vi "DAC_current_values.vi"(1 "FPGA Ref":T1) -> (0 "DAC values":sgl[][](array[numeric]))   [LabVIEW 2013]
uses:
  fpga-bitfile-ref.ctl
  <vilib>/Utility/error.llb/Error Cluster From Error Code.vi
  <vilib>/rvi/errors/niLvFpgaAdjustHostInterfaceError.vi
  <vilib>/rvi/interface/nirviReadWriteControl/nirviReadWriteControl.xnode
  FPGA Bitfiles/fpga-clean1_FPGATarget_FPGAMAINlock-in_FC21E42C.lvbitx
  NiFpgaLv.dll
panel:
  in  "exit":bool
  out "FPGA VI Reference":T1
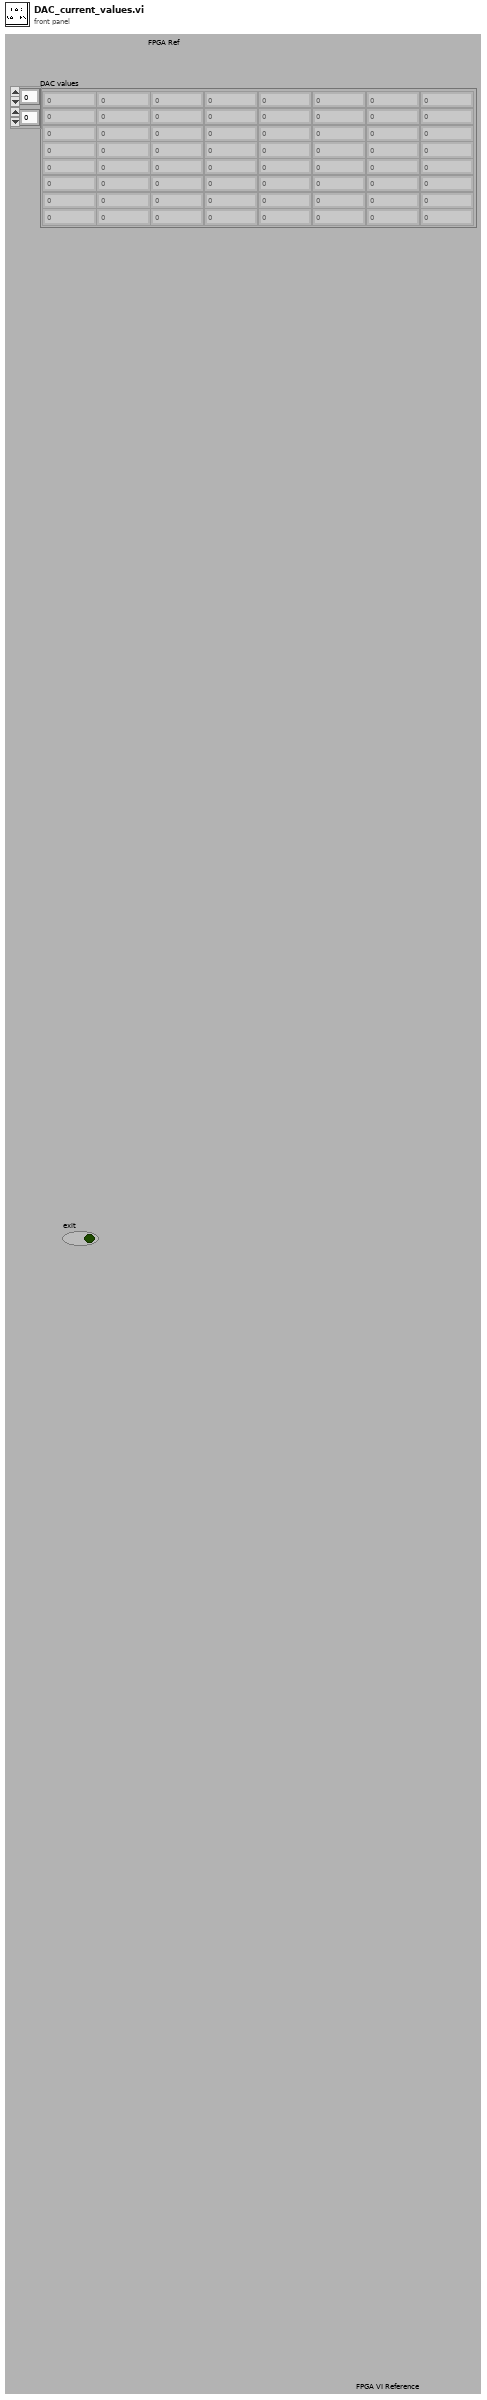
[diagram p1: front panel]
types:
  T1 = typedef "fpga-bitfile-ref.ctl" = refnum<k20>
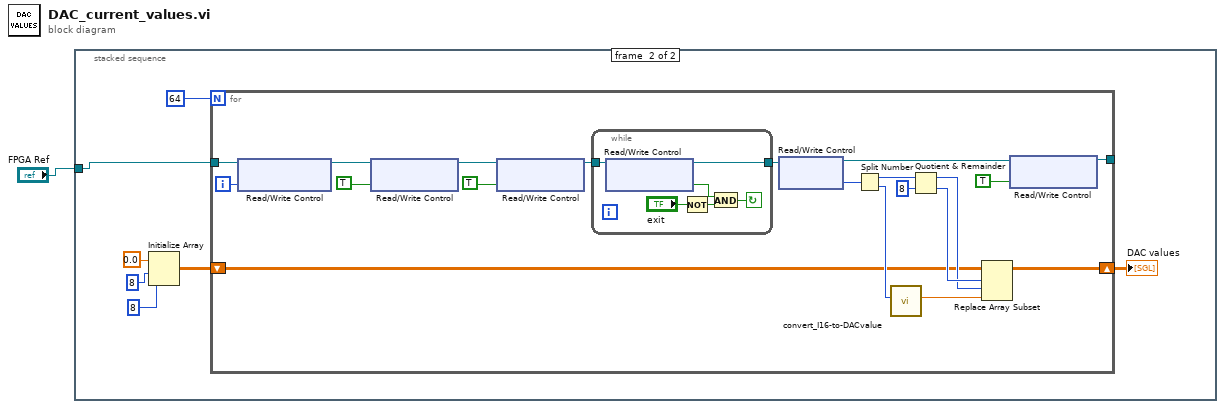
[diagram p0: block diagram]
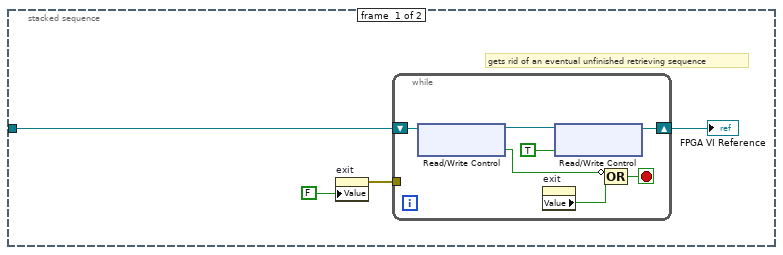
[diagram p2: hidden frame]
diagram:
  n1 = stacked-sequence {
    tunnel: "FPGA Ref" -> [w2 w18]
    frame #0 {
      # "gets rid of an eventual unfinished retrieving sequence"
      n2 = property on="exit" class="Bool (strict)"("Value"=FALSE ("exit")) -> (error out=w4:errorcluster)  [unwired: 2 in, 1 out]
      n3 = while {
        shift-right: [w10] -> w3
        shift-left: w2 -> [w12]
        tunnel: w4 -> [_]
        stop <- w8 stop-if-true
        n4 = xnode "Read/Write Control"("FPGA VI Reference In"=w12) -> ("FPGA VI Reference Out"=w11:T1, "get DAC value"=w7:bool)  [unwired: 1 in, 1 out]
        n5 = property on="exit" class="Bool (strict)"() -> ("Value"=w9:bool)  [unwired: 2 in, 2 out]
        n6 = xnode "Read/Write Control"("FPGA VI Reference In"=w11, "got DAC value"=TRUE) -> ("FPGA VI Reference Out"=w10:T1)  [unwired: 1 in, 1 out]
        n7 = Compound Arithmetic op=OR(invert w7, w9) -> (w8:bool)
      }
      "FPGA VI Reference" <- w3
    }
    frame #1 {
      n8 = Initialize Array(0.0, 8, 8) -> (w13:dbl[][])
      n9 = for {
        N: 64 -> [_]
        tunnel: [w34] -> _
        tunnel: w18 -> [w24]
        shift-right: [w21] -> w17
        shift-left: w13 -> [w20]
        i -> [w29]
        n10 = xnode "Read/Write Control"("FPGA VI Reference In"=w24, "DAC to retrieve"=w29) -> ("FPGA VI Reference Out"=w26:T1)  [unwired: 1 in, 1 out]
        n11 = xnode "Read/Write Control"("FPGA VI Reference In"=w26, "got DAC value"=TRUE ("get DAC values")) -> ("FPGA VI Reference Out"=w25:T1)  [unwired: 1 in, 1 out]
        n12 = xnode "Read/Write Control"("FPGA VI Reference In"=w25, "get DAC value"=TRUE ("get DAC values")) -> ("FPGA VI Reference Out"=w23:T1)  [unwired: 1 in, 1 out]
        n13 = while {
          tunnel: w23 -> [w45]
          tunnel: [w40] -> w39
          stop <- w43 continue-if-true
          n14 = xnode "Read/Write Control"("FPGA VI Reference In"=w45) -> ("FPGA VI Reference Out"=w40:T1, "got DAC value"=w44:bool)  [unwired: 1 in, 1 out]
          n15 = Not(x="exit") -> (.not. x?=w41:bool)
          n16 = And(x=w44, y=w41) -> (x .and. y?=w43:bool)
        }
        n17 = xnode "Read/Write Control"("FPGA VI Reference In"=w39) -> ("FPGA VI Reference Out"=w38:T1, "DAC data"=w36:u32)  [unwired: 1 in, 1 out]
        n18 = Split Number(x=w36) -> (hi(x)=w33:u16, lo(x)=w35:u16)
        n19 = call "convert_I16-to-DACvalue.vi"("DAC Value (I16)"=w35) -> ("DAC value (sgl)"=w30:sgl)  [unwired: 10 out]
        n20 = Quotient & Remainder(x=w33, y=u16 8) -> (x-y*floor(x/y)=w22:u16, floor(x/y)=w31:u16)
        n21 = Replace Array Subset(array=w20, new element=w30, index (row)=w31, index (col)=w22) -> (w21:dbl[][])
        n22 = xnode "Read/Write Control"("FPGA VI Reference In"=w38, "got DAC value"=TRUE) -> ("FPGA VI Reference Out"=w34:T1)  [unwired: 1 in, 1 out]
      }
      "DAC values" <- w17
    }
  }
